vi "Data AcquisitionA.vi"() -> ()   [LabVIEW 2024]
uses:
  <vilib>/Instr/_visa.llb/VISA Configure Serial Port (Instr).vi
panel:
  out "connection information":path
  out "System Number":string
  out "TITLE":string
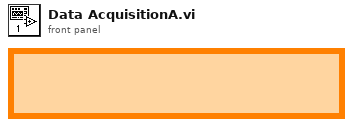
[diagram p1: front panel]
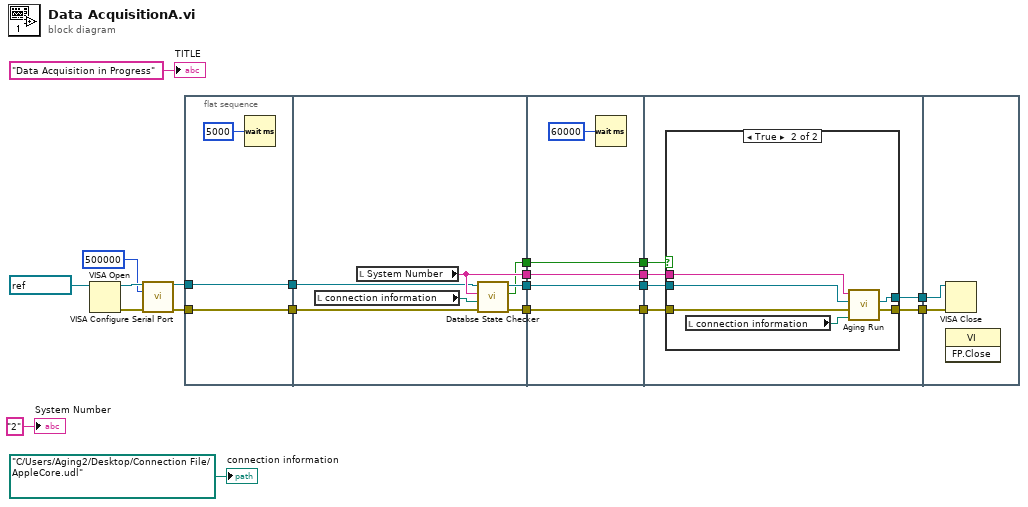
[diagram p0: block diagram]
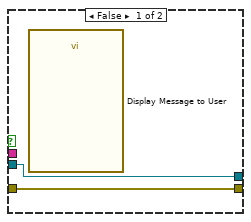
[diagram p2: hidden frame]
diagram:
  n1 = VISA Open(VISA resource name=refnum<visa-resource-name> "COM4") -> (VISA resource name=w20:refnum<visa-resource-name>, error out=w19:errorcluster)  [unwired: 4 in]
  n2 = call-poly "VISA Configure Serial Port"("VISA resource name"=w20, "baud rate (9600)"=u32 500000, "error in (no error)"=w19) -> ("VISA resource name out"=w9:refnum<visa-resource-name>, "error out"=w8:errorcluster)  [unwired: 11 in]
  n3 = flat-sequence {
    tunnel: w8 -> [w23]
    tunnel: w9 -> [w24]
    tunnel: [w24] -> w3
    tunnel: [w23] -> w2
    tunnel: [w31] -> w17
    tunnel: [w29] -> w16
    tunnel: [w28] -> w15
    tunnel: [w27] -> w14
    tunnel: w3 -> [w26]
    tunnel: w2 -> [w30]
    tunnel: [w36] -> w13
    tunnel: w17 -> [w36]
    tunnel: [w35] -> w12
    tunnel: w16 -> [w35]
    tunnel: w15 -> [w34]
    tunnel: [w34] -> w11
    tunnel: [w33] -> w10
    tunnel: w14 -> [w33]
    tunnel: w10 -> [w37]
    tunnel: w11 -> [w38]
    tunnel: w12 -> [w39]
    tunnel: w13 -> [w40]
    tunnel: [w41] -> w5
    tunnel: [w42] -> w4
    tunnel: w5 -> [w52]
    tunnel: w4 -> [w51]
    frame #0 {
      n4 = Wait (ms)(milliseconds to wait=u32 5000) -> ()  [unwired: 1 out]
    }
    frame #1 {
      n5 = local read "connection information"() -> (w25:path)
      n6 = local read "System Number"() -> (w31:string)
      n7 = call "Databse State Checker.vi"("error in (no error)"=w30, "connection information"=w25, "System Number"=w31, "Arduino in"=w26) -> ("error out"=w28:errorcluster, "Database Available?"=w27:bool, "Arduino out"=w29:refnum<visa-resource-name>)  [unwired: 5 in]
    }
    frame #2 {
      n8 = Wait (ms)(milliseconds to wait=u32 60000) -> ()  [unwired: 1 out]
    }
    frame #3 {
      n9 = case shown="True" w37 {
        tunnel: [w44 w50] -> w42
        tunnel: [w43 w49] -> w41
        tunnel: w40 -> [_ w48]
        tunnel: w39 -> [w44 w47]
        tunnel: w38 -> [w43 w46]
        frame False {
          n10 = call "Display Message to User"() -> ()  [unwired: 10 in, 2 out]
        }
        frame True {
          n11 = local read "connection information"() -> (w45:path)
          n12 = call "Aging Run.vi"("UDL"=w45, "error in"=w46, "Arduino"=w47, "System Number"=w48) -> ("error out"=w49:errorcluster, "Arduino"=w50:refnum<visa-resource-name>)  [unwired: 6 in]
        }
      }
    }
    frame #4 {
      n13 = VISA Close(VISA resource name=w51, error in (no error)=w52) -> ()  [unwired: 1 out]
      n14 = invoke class="VI" method="FP.Close"() -> ()  [unwired: 3 in, 3 out]
    }
  }
  "System Number" <- "2" ("substring")
  "TITLE" <- "Data Acquisition in Progress" ("TITLE")
  "connection information" <- path "C:/Users/Aging2/Desktop/Connection File/AppleCore.udl" ("connection information")
